vi "Report_generation.vi"() -> ()   [LabVIEW 2015]
uses:
  <vilib>/Utility/NIReport.llb/NI_report.lvclass
  <vilib>/Utility/NIReport.llb/Append Report Text (str wrap).vi
  <vilib>/Utility/NIReport.llb/NI_ReportGenerationCore.lvlib
  <vilib>/printing/ReportDocExtensions.llb/Append Front Panel Image to Report (path).vi
  <vilib>/printing/OpenHTMLReport.llb/Open HTML Report in Browser (Refnum).vi
  <vilib>/Utility/NIReport.llb/HTML Report Image Alignment.ctl
panel:
  in  "String":string
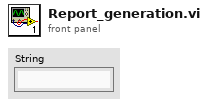
[diagram p1: front panel]
types:
  T1 = typedef "NI_ReportGenerationCore.lvlib/HTML Report Image Alignment.ctl" = enum16{"(default)", "LEFT", "RIGHT", "TOP", "TEXTTOP", "MIDDLE", "ABSMIDDLE", "BASELINE", "BOTTOM", "ABSBOTTOM"}
  T2 = enum16{"Standard Report", "HTML", "Word", "Excel"}
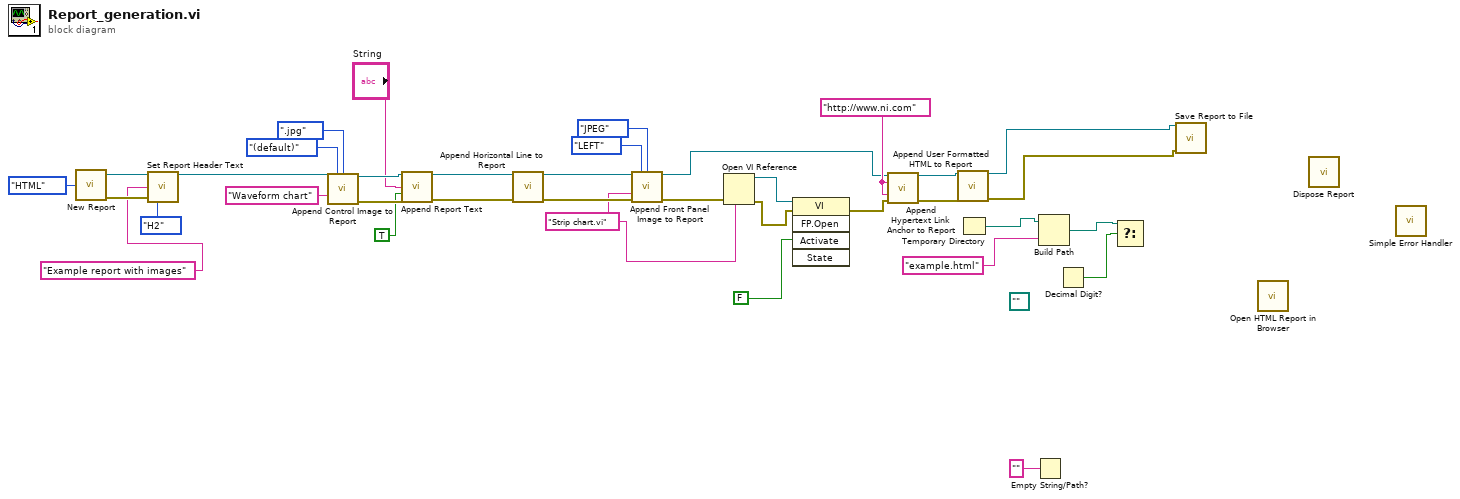
[diagram p0: block diagram]
diagram:
  (unwired) path "" ("f")
  w12 = "http://www.ni.com" ("link text")
  w19 = "Strip chart.vi" ("description")
  n1 = call <vilib>:"New Report.vi"("report type"=T2."HTML") -> ("report out"=w33:refnum<class "NI_report.lvclass">, "error out"=w34:errorcluster)  [unwired: 13 in]
  n2 = call-dynamic "Set Report Header Text.vi"("report in"=w33, "center header text"="Example report with images", "error in (no error)"=w34, "HTML header size"=enum16{"H1", "H2", "H3", "H4", "H5", "H6", "H7"}."H2") -> ("report out"=w30:refnum<class "NI_report.lvclass">)  [unwired: 10 in, 1 out]
  n3 = call-dynamic "Append Control Image to Report.vi"("report in"=w30, "alignment (default)"=HTML_Report_Image_Alignment."(default)", "image file type (.jpg)"=enum16{".jpg", ".png"}.".jpg", "description"="Waveform chart") -> ("report out"=w26:refnum<class "NI_report.lvclass">, "error out"=w25:errorcluster)  [unwired: 8 in, 2 out]
  n4 = call-poly <vilib>:"Append Report Text.vi"("report in"=w26, "text"="String", "append on new line? (F)"=TRUE, "error in (no error)"=w25) -> ("report out"=w24:refnum<class "NI_report.lvclass">, "error out"=w23:errorcluster)  [unwired: 8 in, 2 out]
  n5 = call-dynamic "Append Horizontal Line to Report.vi"("report in"=w24, "error in (no error)"=w23) -> ("report out"=w22:refnum<class "NI_report.lvclass">, "error out"=w21:errorcluster)  [unwired: 12 in]
  n6 = call-poly <vilib>:"Append Front Panel Image to Report.vi"("report in"=w22, "alignment (default)"=HTML_Report_Image_Alignment."LEFT", "image format (jpeg)"=enum32{"PNG", "JPEG", "GIF"}."JPEG", "description"=w19, "error in (no error)"=w21) -> ("report out"=w10:refnum<class "NI_report.lvclass">, "error out"=w20:errorcluster)  [unwired: 6 in, 3 out]
  n7 = Open VI Reference(password ("")=w19, error in (no error)=w20) -> (vi reference=w11:refnum<vi>, error out=w36:errorcluster)  [unwired: 4 in]
  n8 = invoke class="VI" method="FP.Open"(reference=w11, error in=w36, "Activate"=FALSE) -> (error out=w13:errorcluster)  [unwired: 2 in, 4 out]
  n9 = call-dynamic "Append Hypertext Link Anchor to Report.vi"("report in"=w10, "URL of link - href"=w12, "link text"=w12, "error in (no error)"=w13) -> ("report out"=w9:refnum<class "NI_report.lvclass">, "error out"=w8:errorcluster)  [unwired: 8 in, 2 out]
  n10 = call-dynamic "Append User Formatted HTML to Report.vi"("report in"=w9, "error in (no error)"=w8) -> ("report out"=w7:refnum<class "NI_report.lvclass">, "error out"=w6:errorcluster)  [unwired: 12 in]
  n11 = Temporary Directory() -> (w5:path)
  n12 = Empty String/Path?(string/path="") -> ()  [unwired: 1 out]
  n13 = Build Path(base path=w5, name or relative path="example.html") -> (appended path=w2:path)
  n14 = Decimal Digit?() -> (0:w1:bool)  [unwired: 1 in]
  n15 = Select(t=w2, s=w1) -> ()  [unwired: 1 in, 1 out]
  n16 = call-dynamic "Save Report to File.vi"("report in"=w7, "error in (no error)"=w6) -> ()  [unwired: 12 in, 2 out]
  n17 = call-poly <vilib>:"Open HTML Report in Browser.vi"() -> ()  [unwired: 13 in, 3 out]
  n18 = call-dynamic "Dispose Report.vi"() -> ()  [unwired: 15 in, 1 out]
  n19 = call <vilib>:"Simple Error Handler.vi"() -> ()  [unwired: 5 in, 5 out]
